vi "store_InitData_p.vi"(0 "MoAgSy_Host in":refnum<class "MoAgSy_Host.lvclass">, 5 "error in (no error)":errorcluster) -> (19 "error out":errorcluster)   [LabVIEW 2009, in "MoAgSy.lvlib" / "MoAgSy_Host.lvclass"]
doc: "<B>private</B> VI stores init data on disk.\nCalled during host destruction.\nFor next init, the host class object is flattend to string an completely stored in a file.\nIn init, the object is rebuilt and all important settings are assumed.\nStorage path: <working folder>\\initData.bin\n\nF.Berck@gsi.de\nGSI Darmstadt 2009"
uses:
  MoAgSy_Host.lvclass
  MoAgSy_Host.lvclass/MoAgSy_Host.ctl
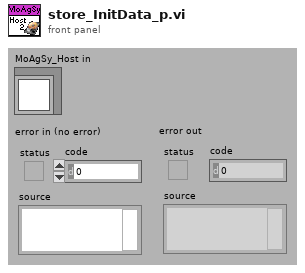
[diagram p1: front panel]
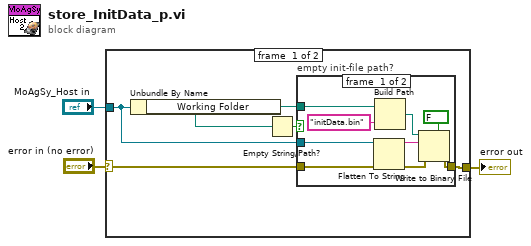
[diagram p0: block diagram]
diagram:
  n1 = case shown="No Error" "error in (no error)" {
    selector: "error in (no error)" -> [w7 w19]
    tunnel: [w6 w19] -> w2
    tunnel: "MoAgSy_Host in" -> [w8 _]
    frame #0 {
      n2 = Unbundle By Name(w8) -> ("Working Folder"=w5:path)
      n3 = Empty String/Path?(string/path=w5) -> (empty?=w4:bool)
      n4 = case "empty init-file path?" shown="False" w4 {
        tunnel: w8 -> [w17 _]
        tunnel: w7 -> [w16 w18]
        tunnel: w5 -> [w12 _]
        tunnel: [w13 w18] -> w6
        frame #0 {
          n5 = Flatten To String(anything=w17, error in (no error)=w16) -> (data string=w15:string, error out=w14:errorcluster)  [unwired: 3 out]
          n6 = Build Path(base path=w12, name or relative path="initData.bin") -> (appended path=w10:path)
          n7 = Write to Binary File(file (use dialog)=w10, data=w15, error in=w14, 5:FALSE ("prepend array or string size? (T)")) -> (error out=w13:errorcluster)  [unwired: 4 out]
        }
        frame #1 {
        }
      }
    }
    frame #1 {
    }
  }
  "error out" <- w2
